vi "Chair Plugin.vi"(10 "DC File":path, 11 "Data IN":T3={"Impulse Positions"=[{"Start"=3107, "End"=3217, "Impulse Plane"=enum."Yaw", "Impulse Direction +ve?"=FALSE, "Time offset"=0, "Amplitude offset"=0.0}, {"Start"=3536, "End"=3646, "Impulse Plane"=enum."Yaw", "Impulse Direction +ve?"=FALSE, "Time offset"=0, "Amplitude offset"=0.0}, {"Start"=4980, "End"=5091, "Impulse Plane"=enum."Yaw", "Impulse Direction +ve?"=TRUE, "Time offset"=0, "Amplitude offset"=0.0}, {"Start"=5459, "End"=5570, "Impulse Plane"=enum."Yaw", "Impulse Direction +ve?"=TRUE, "Time offset"=0, "Amplitude offset"=0.0}, {"Start"=6047, "End"=6157, "Impulse Plane"=enum."Yaw", "Impulse Direction +ve?"=TRUE, "Time offset"=0, "Amplitude offset"=0.0}, {"Start"=6820, "End"=6931, "Impulse Plane"=enum."Yaw", "Impulse Direction +ve?"=TRUE, "Time offset"=0, "Amplitude offset"=0.0}, {"Start"=7337, "End"=7447, "Impulse Plane"=enum."Yaw", "Impulse Direction +ve?"=FALSE, "Time offset"=0, "Amplitude offset"=0.0}, {"Start"=7787, "End"=7897, "Impulse Plane"=enum."Yaw", "Impulse Direction +ve?"=FALSE, "Time offset"=0, "Amplitude offset"=0.0}, {"Start"=8584, "End"=8694, "Impulse Plane"=enum."Yaw", "Impulse Direction +ve?"=FALSE, "Time offset"=0, "Amplitude offset"=0.0}, {"Start"=10739, "End"=10849, "Impulse Plane"=enum."Yaw", "Impulse Direction +ve?"=TRUE, "Time offset"=0, "Amplitude offset"=0.0}, {"Start"=13129, "End"=13240, "Impulse Plane"=enum."Yaw", "Impulse Direction +ve?"=FALSE, "Time offset"=0, "Amplitude offset"=0.0}, {"Start"=13282, "End"=13390, "Impulse Plane"=enum."Yaw", "Impulse Direction +ve?"=FALSE, "Time offset"=0, "Amplitude offset"=0.0}, {"Start"=14766, "End"=14875, "Impulse Plane"=enum."Yaw", "Impulse Direction +ve?"=TRUE, "Time offset"=0, "Amplitude offset"=0.0}, {"Start"=15667, "End"=15777, "Impulse Plane"=enum."Yaw", "Impulse Direction +ve?"=FALSE, "Time offset"=0, "Amplitude offset"=0.0}], "No. Imp"=8, "Parameter Time Series"=[{"time offset"=0.0, "Offset"=0.0, "Gain"=1.0, "inverse"=FALSE, "filter data"=FALSE, "dots"=FALSE, "interpolate"=FALSE, "List 1"=1, "Color Box"=65295, "Boolean"=TRUE}, {"time offset"=0.0, "Offset"=0.0, "Gain"=1.0, "inverse"=FALSE, "filter data"=FALSE, "dots"=FALSE, "interpolate"=FALSE, "List 1"=13, "Color Box"=29695, "Boolean"=TRUE}, {"time offset"=0.0, "Offset"=0.0, "Gain"=1.0, "inverse"=FALSE, "filter data"=FALSE, "dots"=FALSE, "interpolate"=FALSE, "List 1"=21, "Color Box"=16711680, "Boolean"=TRUE}], "Parameter Impuls Series"=[{"Color"=4652800, "Visible"=TRUE, "Channel"=1, "Invert"=FALSE, "Desaccade"=FALSE, "Offset"=0.0, "Gain"=1.0}, {"Color"=16860, "Visible"=TRUE, "Channel"=13, "Invert"=FALSE, "Desaccade"=FALSE, "Offset"=0.0, "Gain"=1.0}, {"Color"=16711680, "Visible"=TRUE, "Channel"=21, "Invert"=FALSE, "Desaccade"=FALSE, "Offset"=0.0, "Gain"=1.0}], "Experiment Parameters"={"Freq"=nan, "Vel"=-1, "Acc"=0, "Stimulus"="Head Impulse -Horizontal"}, "Autosort File"=refnum, "Data File"={"Data Channels"=array22x16587[364914 elements], "Sample Rate"=221, "Channel List"=["-", "Hz Velocity-in-Head", "-", "Hy Velocity-in-Head", "-", "Hx Velocity-in-Head", "-", "-", "-", "-", "-", "Lx Velocity-in-Head", "Ly Velocity-in-Head", "Lz Velocity-in-Head", "-", "-", "-", "-", "-", "Rx Velocity-in-Head", "Ry Velocity-in-Head", "Rz Velocity-in-Head"]}, "Experiment data path"=path "C:/Users/w.figtree/Desktop/Test Data/D246 - Lyndall Westman", "Image data path"=path "C:/Users/w.figtree/Desktop", "LVS data path"=path "/Macintosh HD/Users/patrick/Studium/Diploma Thesis/Data Analysis", "Raw copy path"=path "/Macintosh HD/Users/patrick/Studium/Diploma Thesis/Data Analysis", "filename"="p00195s001e016c001t001.mat", "desaccading parameters"={"Tolerance"=3, "Acc Range"=7000.0, "Sample Rate"=221, "Impulse Plane 2"=enum."Yaw", "Impulse dir"=TRUE}, "Experiment Parameters 2"={"Subject"="Westman Lyndall", "Strain"="(4a) _ OptKin_50_left", "Rotation plane"="", "Experimenter"="Musterdoc", "Trial"=0.0, "Time"=0.0}, "Excel"={"Excel._Application"=refnum, "Use Excel"=TRUE, "Worksheet SINE"=refnum, "Row SINE"=0, "Worksheet TRANS"=refnum, "Row TRANS"=0}, "Session Config File"=refnum, "Autosort Parameter Set"=10, "EMA Version"="EMA 2011b", "desacc "={"Threshold 1 [Acc]"=7000.0, "Threshold 2 [% of TH1]"=60, "tolerance"=3, "Search WD "=0.1, " always use TH2"=FALSE, "Range"=3.0, "Max time"=120.0, "Min time"=20.0, "Velocity Threshold"=150}, "Cycle Nr for Saccades"={"POS"=0, "NEG"=6}, "calibration name"="No file selected"} {"Parameter Time Series"."time offset" format="%.3f"; "Parameter Time Series"."Gain" format="%.1f"; "Parameter Time Series"."Offset" format="%.1f"; "Parameter Time Series"."List 1" items=["Motor-Pos", "Motor-Vel", "Lx Position-in-Head", "Ly Position-in-Head", "Lz Position-in-Head", "Lx Velocity-in-Head", "Ly Velocity-in-Head", "Lz Velocity-in-Head", "Ll Velocity-in-Head", "Lr Velocity-in-Head", "Lx Accel-in-Head", "Ly Accel-in-Head", "Lz Accel-in-Head", "Rx Position-in-Head", "Ry Position-in-Head", "Rz Position-in-Head", "Rx Velocity-in-Head", "Ry Velocity-in-Head", "Rz Velocity-in-Head", "Rl Velocity-in-Head", "Rr Velocity-in-Head", "Rx Accel-in-Head", "Ry Accel-in-Head", "Rz Accel-in-Head", "Global Trigger", "", "", ""]; "Parameter Impuls Series"."Gain" format="%.1f"; "Parameter Impuls Series"."Offset" format="%.1f"}) -> (2 "Cancelled":bool=TRUE, 3 "Data OUT":T3={"Impulse Positions"=[{"Start"=3107, "End"=3217, "Impulse Plane"=enum."Yaw", "Impulse Direction +ve?"=FALSE, "Time offset"=0, "Amplitude offset"=0.0}, {"Start"=3536, "End"=3646, "Impulse Plane"=enum."Yaw", "Impulse Direction +ve?"=FALSE, "Time offset"=0, "Amplitude offset"=0.0}, {"Start"=4980, "End"=5091, "Impulse Plane"=enum."Yaw", "Impulse Direction +ve?"=TRUE, "Time offset"=0, "Amplitude offset"=0.0}, {"Start"=5459, "End"=5570, "Impulse Plane"=enum."Yaw", "Impulse Direction +ve?"=TRUE, "Time offset"=0, "Amplitude offset"=0.0}, {"Start"=6047, "End"=6157, "Impulse Plane"=enum."Yaw", "Impulse Direction +ve?"=TRUE, "Time offset"=0, "Amplitude offset"=0.0}, {"Start"=6820, "End"=6931, "Impulse Plane"=enum."Yaw", "Impulse Direction +ve?"=TRUE, "Time offset"=0, "Amplitude offset"=0.0}, {"Start"=7337, "End"=7447, "Impulse Plane"=enum."Yaw", "Impulse Direction +ve?"=FALSE, "Time offset"=0, "Amplitude offset"=0.0}, {"Start"=7787, "End"=7897, "Impulse Plane"=enum."Yaw", "Impulse Direction +ve?"=FALSE, "Time offset"=0, "Amplitude offset"=0.0}, {"Start"=8584, "End"=8694, "Impulse Plane"=enum."Yaw", "Impulse Direction +ve?"=FALSE, "Time offset"=0, "Amplitude offset"=0.0}, {"Start"=10739, "End"=10849, "Impulse Plane"=enum."Yaw", "Impulse Direction +ve?"=TRUE, "Time offset"=0, "Amplitude offset"=0.0}, {"Start"=13129, "End"=13240, "Impulse Plane"=enum."Yaw", "Impulse Direction +ve?"=FALSE, "Time offset"=0, "Amplitude offset"=0.0}, {"Start"=13282, "End"=13390, "Impulse Plane"=enum."Yaw", "Impulse Direction +ve?"=FALSE, "Time offset"=0, "Amplitude offset"=0.0}, {"Start"=14766, "End"=14875, "Impulse Plane"=enum."Yaw", "Impulse Direction +ve?"=TRUE, "Time offset"=0, "Amplitude offset"=0.0}, {"Start"=15667, "End"=15777, "Impulse Plane"=enum."Yaw", "Impulse Direction +ve?"=FALSE, "Time offset"=0, "Amplitude offset"=0.0}], "No. Imp"=8, "Parameter Time Series"=[{"time offset"=0.0, "Offset"=0.0, "Gain"=1.0, "inverse"=FALSE, "filter data"=FALSE, "dots"=FALSE, "interpolate"=FALSE, "List 1"=1, "Color Box"=65295, "Boolean"=TRUE}, {"time offset"=0.0, "Offset"=0.0, "Gain"=1.0, "inverse"=FALSE, "filter data"=FALSE, "dots"=FALSE, "interpolate"=FALSE, "List 1"=13, "Color Box"=29695, "Boolean"=TRUE}, {"time offset"=0.0, "Offset"=0.0, "Gain"=1.0, "inverse"=FALSE, "filter data"=FALSE, "dots"=FALSE, "interpolate"=FALSE, "List 1"=21, "Color Box"=16711680, "Boolean"=TRUE}], "Parameter Impuls Series"=[{"Color"=4652800, "Visible"=TRUE, "Channel"=1, "Invert"=FALSE, "Desaccade"=FALSE, "Offset"=0.0, "Gain"=1.0}, {"Color"=16860, "Visible"=TRUE, "Channel"=13, "Invert"=FALSE, "Desaccade"=FALSE, "Offset"=0.0, "Gain"=1.0}, {"Color"=16711680, "Visible"=TRUE, "Channel"=21, "Invert"=FALSE, "Desaccade"=FALSE, "Offset"=0.0, "Gain"=1.0}], "Experiment Parameters"={"Freq"=nan, "Vel"=-1, "Acc"=0, "Stimulus"="Head Impulse -Horizontal"}, "Autosort File"=refnum, "Data File"={"Data Channels"=array22x16587[364914 elements], "Sample Rate"=221, "Channel List"=["-", "Hz Velocity-in-Head", "-", "Hy Velocity-in-Head", "-", "Hx Velocity-in-Head", "-", "-", "-", "-", "-", "Lx Velocity-in-Head", "Ly Velocity-in-Head", "Lz Velocity-in-Head", "-", "-", "-", "-", "-", "Rx Velocity-in-Head", "Ry Velocity-in-Head", "Rz Velocity-in-Head"]}, "Experiment data path"=path "C:/Users/w.figtree/Desktop/Test Data/D246 - Lyndall Westman", "Image data path"=path "C:/Users/w.figtree/Desktop", "LVS data path"=path "/Macintosh HD/Users/patrick/Studium/Diploma Thesis/Data Analysis", "Raw copy path"=path "/Macintosh HD/Users/patrick/Studium/Diploma Thesis/Data Analysis", "filename"="p00195s001e016c001t001.mat", "desaccading parameters"={"Tolerance"=3, "Acc Range"=7000.0, "Sample Rate"=221, "Impulse Plane 2"=enum."Yaw", "Impulse dir"=TRUE}, "Experiment Parameters 2"={"Subject"="Westman Lyndall", "Strain"="(4a) _ OptKin_50_left", "Rotation plane"="", "Experimenter"="Musterdoc", "Trial"=0.0, "Time"=0.0}, "Excel"={"Excel._Application"=refnum, "Use Excel"=TRUE, "Worksheet SINE"=refnum, "Row SINE"=0, "Worksheet TRANS"=refnum, "Row TRANS"=0}, "Session Config File"=refnum, "Autosort Parameter Set"=10, "EMA Version"="EMA 2011b", "desacc "={"Threshold 1 [Acc]"=7000.0, "Threshold 2 [% of TH1]"=60, "tolerance"=3, "Search WD "=0.1, " always use TH2"=FALSE, "Range"=3.0, "Max time"=120.0, "Min time"=20.0, "Velocity Threshold"=150}, "Cycle Nr for Saccades"={"POS"=0, "NEG"=6}, "calibration name"="No file selected"} {"Parameter Time Series"."time offset" format="%.3f"; "Parameter Time Series"."Gain" format="%.1f"; "Parameter Time Series"."Offset" format="%.1f"; "Parameter Time Series"."List 1" items=["Motor-Pos", "Motor-Vel", "Lx Position-in-Head", "Ly Position-in-Head", "Lz Position-in-Head", "Lx Velocity-in-Head", "Ly Velocity-in-Head", "Lz Velocity-in-Head", "Ll Velocity-in-Head", "Lr Velocity-in-Head", "Lx Accel-in-Head", "Ly Accel-in-Head", "Lz Accel-in-Head", "Rx Position-in-Head", "Ry Position-in-Head", "Rz Position-in-Head", "Rx Velocity-in-Head", "Ry Velocity-in-Head", "Rz Velocity-in-Head", "Rl Velocity-in-Head", "Rr Velocity-in-Head", "Rx Accel-in-Head", "Ry Accel-in-Head", "Rz Accel-in-Head", "Global Trigger", "", "", ""]; "Parameter Impuls Series"."Gain" format="%.1f"; "Parameter Impuls Series"."Offset" format="%.1f"})   [LabVIEW 2016]
uses:
  core/type-defs/TD_Statemachine-Data.ctl
  core/type-defs/TD_Time Series.ctl
  core/type-defs/TD_Impulse Parameter.ctl
  <vilib>/Utility/file.llb/Read From Spreadsheet File (DBL).vi
  <userlib>/_OpenG.lib/array/array.llb/Reverse 2D Array (DBL)__ogtk.vi
  core/core.lvlib
panel:
  in  "stop 2":bool
  in  "process":bool
  in  "Tab Control":enum32{"Time Plot", "Impuls Plot"}(tab)
  in  "Plot Selection":T1=[{"time offset"=0.0, "Offset"=0.0, "Gain"=1.0, "inverse"=FALSE, "filter data"=FALSE, "dots"=FALSE, "interpolate"=FALSE, "List 1"=1, "Color Box"=65309, "Boolean"=TRUE}, {"time offset"=0.0, "Offset"=0.0, "Gain"=1.0, "inverse"=FALSE, "filter data"=FALSE, "dots"=FALSE, "interpolate"=FALSE, "List 1"=8, "Color Box"=29695, "Boolean"=TRUE}, {"time offset"=0.0, "Offset"=0.0, "Gain"=1.0, "inverse"=FALSE, "filter data"=FALSE, "dots"=FALSE, "interpolate"=FALSE, "List 1"=14, "Color Box"=16711680, "Boolean"=TRUE}] {"time offset" format="%.3f"; "Gain" format="%.1f"; "Offset" format="%.1f"; "List 1" items=["Chair Position", "Chair Velocity", "Light Off/On", "Lx Position-in-Head", "Ly Position-in-Head", "Lz Position-in-Head", "Lx Velocity-in-Head", "Ly Velocity-in-Head", "Lz Velocity-in-Head", "Rx Position-in-Head", "Ry Position-in-Head", "Rz Position-in-Head", "Rx Velocity-in-Head", "Ry Velocity-in-Head", "Rz Velocity-in-Head"]}
  in  "Plot Selection 2":T2=[{"Color"=4652800, "Visible"=TRUE, "Channel"=1, "Invert"=FALSE, "Desaccade"=FALSE, "Offset"=0.0, "Gain"=1.0}, {"Color"=29695, "Visible"=TRUE, "Channel"=8, "Invert"=FALSE, "Desaccade"=FALSE, "Offset"=0.0, "Gain"=1.0}, {"Color"=16711680, "Visible"=TRUE, "Channel"=14, "Invert"=FALSE, "Desaccade"=FALSE, "Offset"=0.0, "Gain"=1.0}] {"Gain" format="%.1f"; "Offset" format="%.1f"; "Channel" items=["Chair Position", "Chair Velocity", "Light Off/On", "Lx Position-in-Head", "Ly Position-in-Head", "Lz Position-in-Head", "Lx Velocity-in-Head", "Ly Velocity-in-Head", "Lz Velocity-in-Head", "Rx Position-in-Head", "Ry Position-in-Head", "Rz Position-in-Head", "Rx Velocity-in-Head", "Ry Velocity-in-Head", "Rz Velocity-in-Head"]}
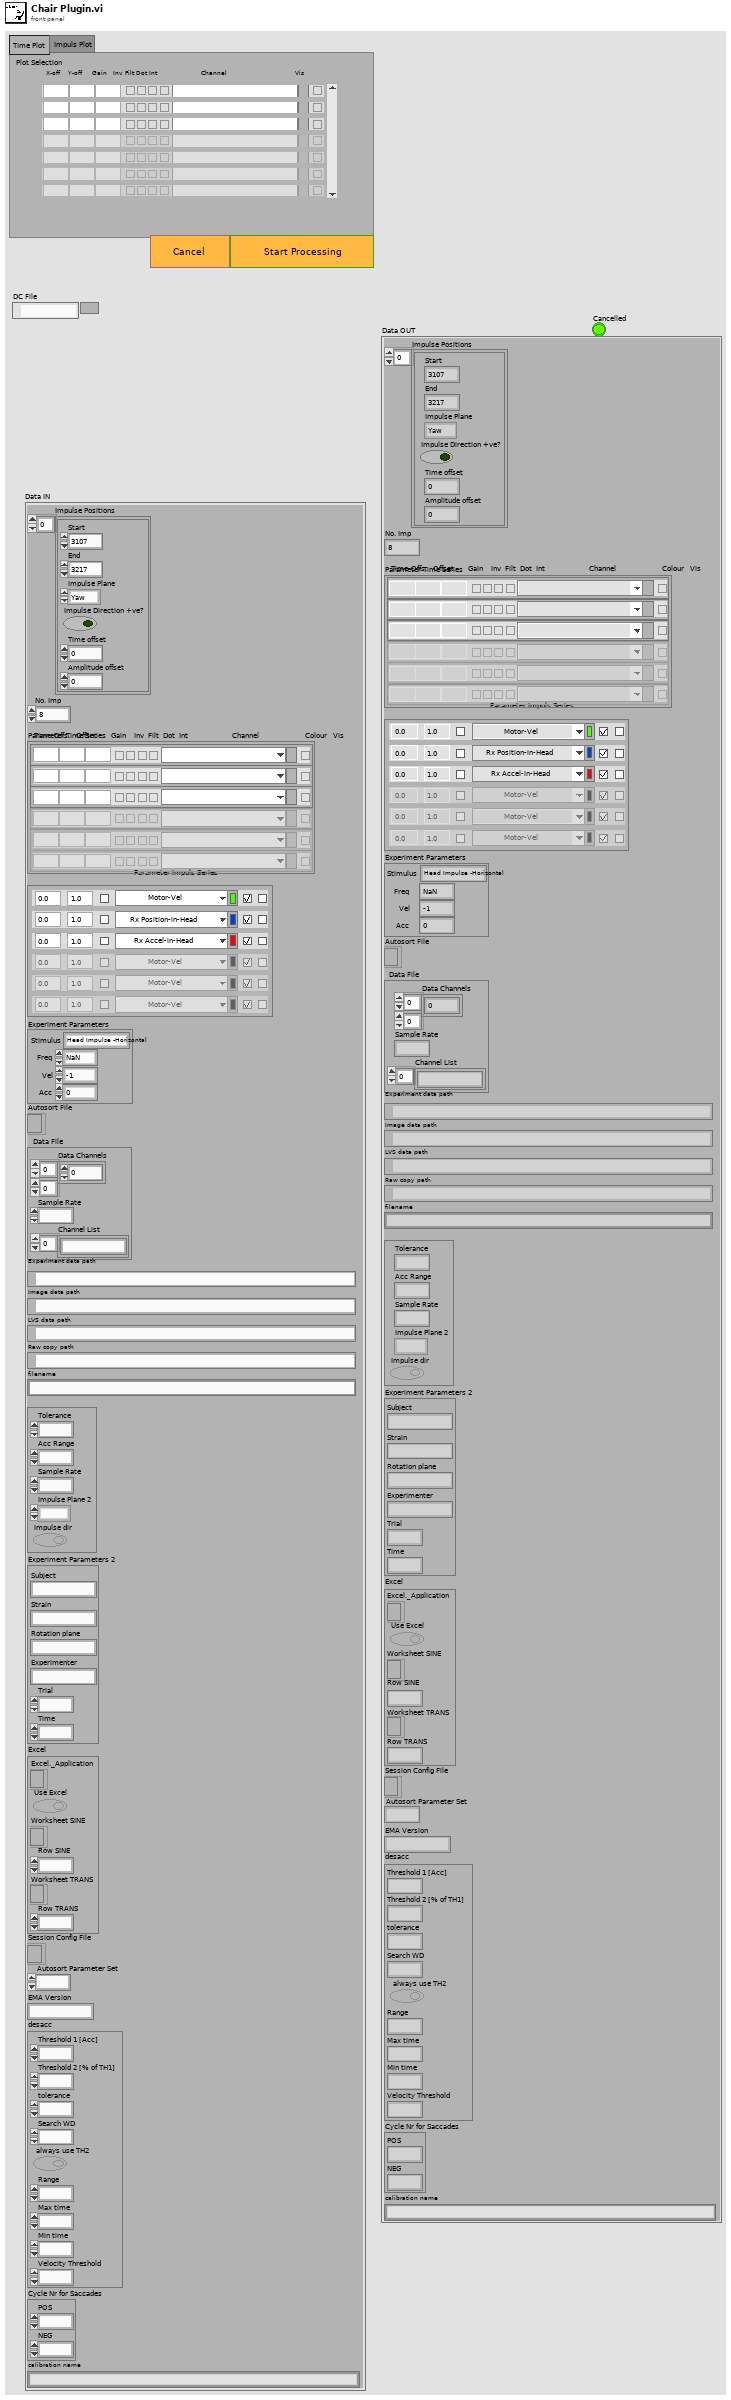
[diagram p1: front panel]
types:
  T1 = typedef "core.lvlib/TD_Time Series.ctl" = cluster{"time offset":dbl, "Offset":dbl, "Gain":dbl, "inverse":bool, "filter data":bool, "dots":bool, "interpolate":bool, "List 1":u16, "Color Box":u32, "Boolean":bool}[]
  T2 = typedef "core.lvlib/TD_Impulse Parameter.ctl" = cluster{"Color":u32, "Visible":bool, "Channel":u16, "Invert":bool, "Desaccade":bool, "Offset":dbl, "Gain":dbl}[]
  T3 = typedef "core.lvlib/TD_Statemachine-Data.ctl" = cluster{"Impulse Positions":cluster{"Start":i32, "End":i32, "Impulse Plane":enum16{"Other", "Yaw", "Pitch", "Roll", "LARP", "RALP"}, "Impulse Direction +ve?":bool, "Time offset":i32, "Amplitude offset":dbl}[], "No. Imp":i32, "Parameter Time Series":T1, "Parameter Impuls Series":T2, "Experiment Parameters":cluster{"Freq":dbl, "Vel":i32, "Acc":i32, "Stimulus":string}, "Autosort File":refnum<file>, "Data File":cluster{"Data Channels":dbl[][], "Sample Rate":i32, "Channel List":string[]}, "Experiment data path":path, "Image data path":path, "LVS data path":path, "Raw copy path":path, "filename":string, "desaccading parameters":cluster{"Tolerance":i32, "Acc Range":dbl, "Sample Rate":i32, "Impulse Plane 2":enum16{"Other", "Yaw", "Pitch", "Roll", "LARP", "RALP"}, "Impulse dir":bool}, "Experiment Parameters 2":cluster{"Subject":string, "Strain":string, "Rotation plane":string, "Experimenter":string, "Trial":dbl, "Time":dbl}, "Excel":cluster{"Excel._Application":refnum<k7>, "Use Excel":bool, "Worksheet SINE":refnum<k7>, "Row SINE":i32, "Worksheet TRANS":refnum<k7>, "Row TRANS":i32}, "Session Config File":refnum<file>, "Autosort Parameter Set":i32, "EMA Version":string, "desacc ":cluster{"Threshold 1 [Acc]":dbl, "Threshold 2 [% of TH1]":i32, "tolerance":i32, "Search WD ":dbl, " always use TH2":bool, "Range":dbl, "Max time":dbl, "Min time":dbl, "Velocity Threshold":i32}, "Cycle Nr for Saccades":cluster{"POS":i32, "NEG":i32}, "calibration name":string}
  T4 = cluster{"File Path":path, "Raw Data":sgl[][], "Sample Rate":i32}
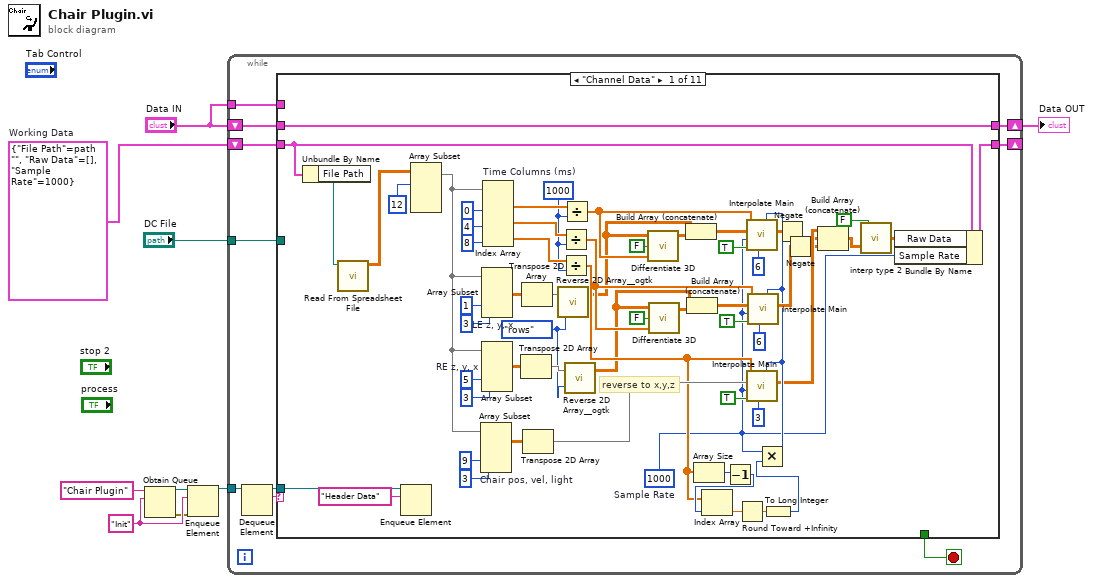
[diagram p0: block diagram]
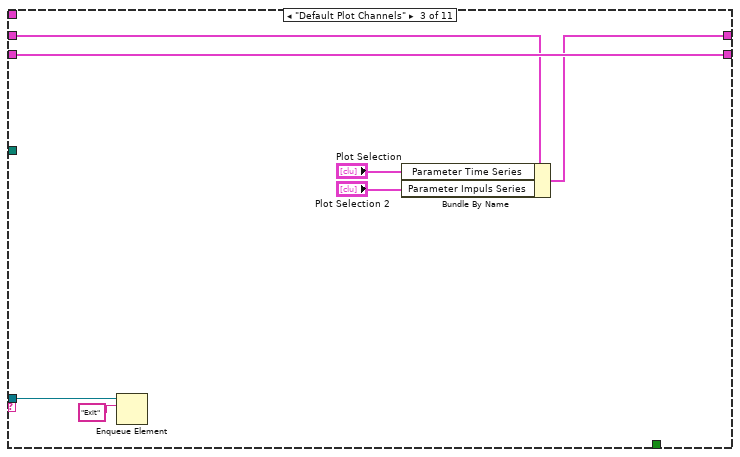
[diagram p3: hidden frame]
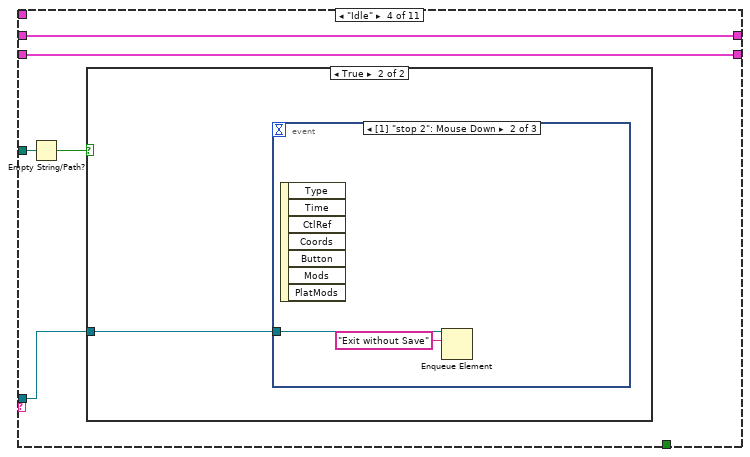
[diagram p4: hidden frame]
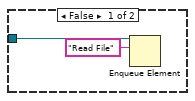
[diagram p5: hidden frame]
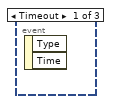
[diagram p6: hidden frame]
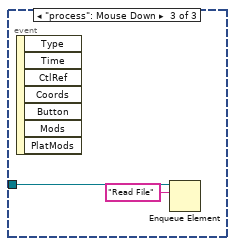
[diagram p7: hidden frame]
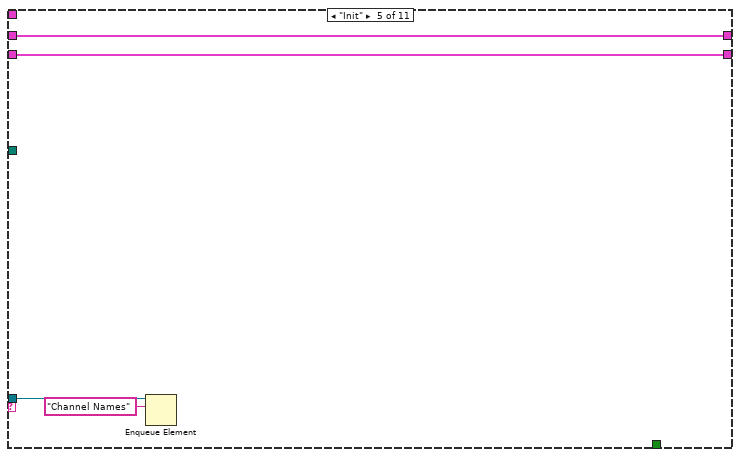
[diagram p8: hidden frame]
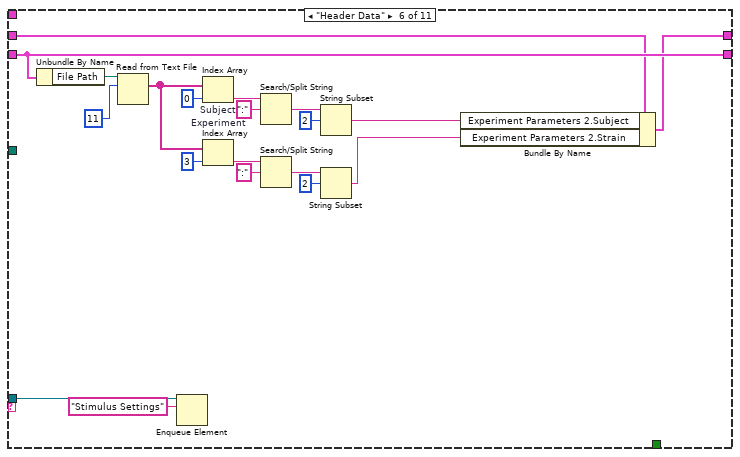
[diagram p9: hidden frame]
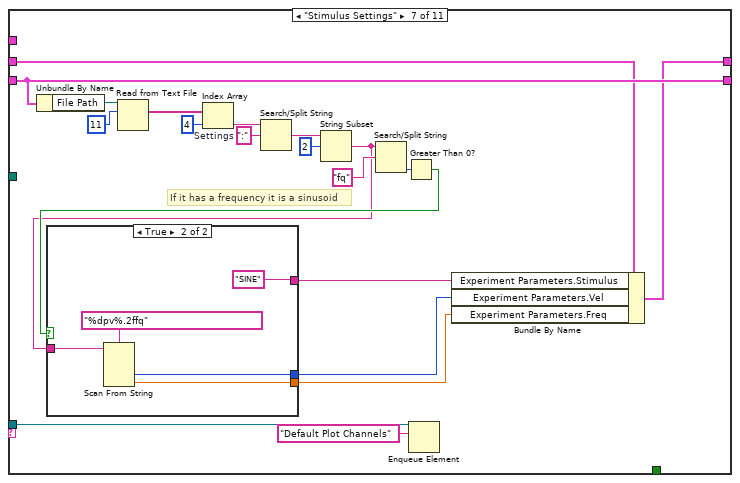
[diagram p10: hidden frame]
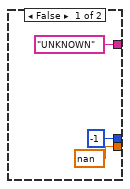
[diagram p11: hidden frame]
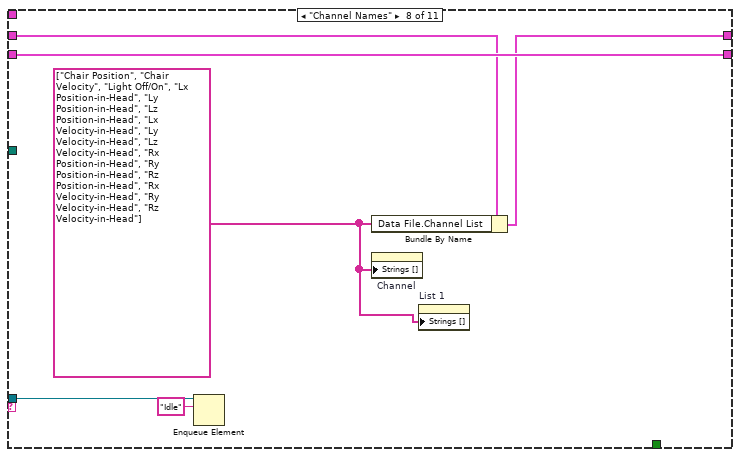
[diagram p12: hidden frame]
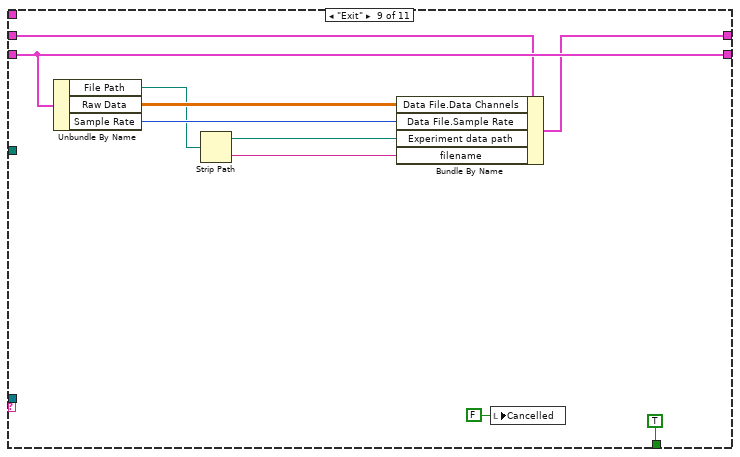
[diagram p13: hidden frame]
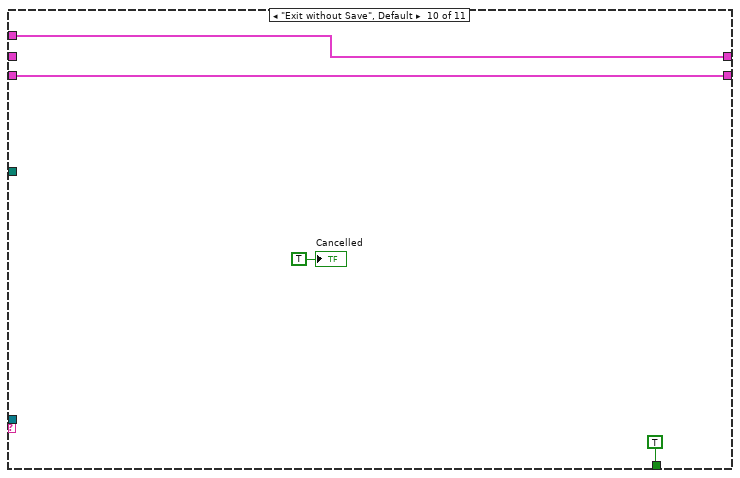
[diagram p14: hidden frame]
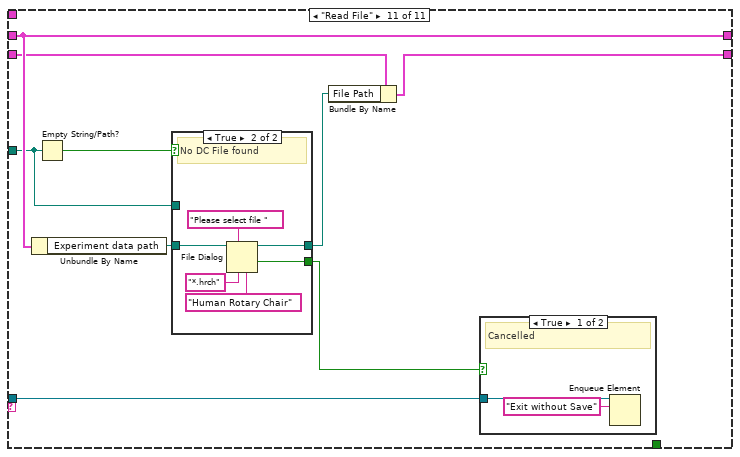
[diagram p15: hidden frame]
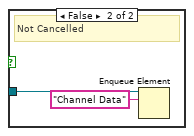
[diagram p16: hidden frame]
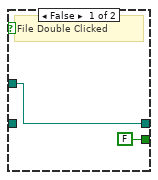
[diagram p17: hidden frame]
diagram:
  w2 = T4 {"File Path"=path "", "Raw Data"=[], "Sample Rate"=1000}  # Working Data
  w7 = "Init" ("name (unnamed)")
  n1 = Obtain Queue(name (unnamed)="Chair Plugin", element data type=w7) -> (queue out=w8:refnum<queue>, error out=w6:errorcluster)  [unwired: 3 in, 1 out]
  n2 = Enqueue Element(queue=w8, element=w7, error in (no error)=w6) -> (queue out=w5:refnum<queue>)  [unwired: 1 in, 2 out]
  n3 = while {
    tunnel: w5 -> [w19]
    tunnel: "DC File" -> [w15]
    shift-right: [w16] -> w4
    shift-left: "Data IN" -> [w17]
    shift-right: [w13] -> _
    shift-left: w2 -> [w14]
    tunnel: "Data IN" -> [w10]
    stop <- w11 stop-if-true
    n4 = Dequeue Element(queue=w19) -> (queue out=w12:refnum<queue>, element=w18:string)  [unwired: 2 in, 2 out]
    n5 = case shown="\"Channel Data\"" w18 {
      tunnel: w17 -> [w80 w82 w88 w94 w105 w117 w137 w158 w165 _ w181]
      tunnel: [w80 w82 w87 w94 w105 w116 w136 w157 w164 w172 w181] -> w16
      tunnel: w15 -> [_ _ _ w92 _ _ _ _ _ _ w179]
      tunnel: w14 -> [w35 w81 w89 w93 w104 w125 w145 w159 w168 w171 w177]
      tunnel: [w34 w81 w89 w93 w104 w125 w145 w159 w168 w171 w176] -> w13
      tunnel: w12 -> [w32 _ w84 w90 w103 w107 w127 w156 _ _ w175]
      tunnel: [_ _ _ _ _ _ _ _ TRUE TRUE _] -> w11
      tunnel: w10 -> [_ _ _ _ _ _ _ _ _ w172 _]
      frame "Channel Data" {
        w23 = enum16{"rows", "columns"}."rows" ("by rows or columns (rows)")
        w40 = 1000 ("Sample Rate")
        w33 = 1000  # Sample Rate
        # "reverse to x,y,z"
        n6 = Unbundle By Name(w35) -> ("File Path"=w36:path)
        n7 = call-poly <vilib>:"Read From Spreadsheet File.vi"("file path (dialog if empty)"=w36) -> ("all rows"=w78:dbl[][])  [unwired: 6 in, 4 out]
        n8 = Enqueue Element(queue=w32, element="Header Data") -> ()  [unwired: 2 in, 3 out]
        n9 = Array Subset(array=w78, index (row)=12 ("index")) -> (w63:dbl[][])  [unwired: 3 in]
        n10 = Array Subset "Chair pos, vel, light"(array=w63, index (col)=9 ("index"), length (col)=3 ("length")) -> (w46:dbl[][])  [unwired: 2 in]
        n11 = Array Subset "LE z, y, x"(array=w63, index (col)=1 ("index"), length (col)=3 ("length")) -> (w71:dbl[][])  [unwired: 2 in]
        n12 = Array Subset "RE z, y, x"(array=w63, index (col)=5 ("index"), length (col)=3 ("length")) -> (w66:dbl[][])  [unwired: 2 in]
        n13 = Index Array "Time Columns (ms)"(array=w63, index (col) #1=0 ("index (row)"), index (col) #2=4 ("index (row)"), index (col) #3=8 ("index (row)")) -> (element #1=w43:dbl[], element #2=w42:dbl[], element #3=w41:dbl[])  [unwired: 3 in]
        n14 = Transpose 2D Array(2D array=w66) -> (transposed array=w25:dbl[][])
        n15 = Transpose 2D Array(2D array=w71) -> (transposed array=w27:dbl[][])
        n16 = Transpose 2D Array(2D array=w46) -> (transposed array=w45:dbl[][])
        n17 = call-poly <userlib>:"Reverse 2D Array__ogtk.vi"("by rows or columns (rows)"=w23, "Array"=w27) -> ("Reversed Array"=w26:dbl[][])  [unwired: 1 in]
        n18 = Divide(x=w42, y=w40) -> (x/y=w38:dbl[])
        n19 = Divide(x=w41, y=w40) -> (x/y=w39:dbl[])
        n20 = Divide(x=w43, y=w40) -> (x/y=w37:dbl[])
        n21 = call-poly <userlib>:"Reverse 2D Array__ogtk.vi"("by rows or columns (rows)"=w23, "Array"=w25) -> ("Reversed Array"=w24:dbl[][])  [unwired: 1 in]
        n22 = call "Differentiate 3D.vi"("Timebase"=w37, "Fixed Sample Rate"=FALSE, "Data (in)"=w26) -> ("Data (differentiated)"=w72:dbl[][])  [unwired: 2 in]
        n23 = call "Differentiate 3D.vi"("Timebase"=w38, "Fixed Sample Rate"=FALSE, "Data (in)"=w24) -> ("Data (differentiated)"=w67:dbl[][])  [unwired: 2 in]
        n24 = Build Array (concatenate)(w26, w72) -> (w70:dbl[][])
        n25 = Build Array (concatenate)(w24, w67) -> (w69:dbl[][])
        n26 = Array Size(array=w39) -> (size(s)=w56:i32)
        n27 = Decrement(x=w56) -> (x-1=w44:i32)
        n28 = Index Array(array=w39, index=w44) -> (element=w55:dbl)
        n29 = Round Toward +Infinity(x=w55) -> (ceil(x): smallest int >= x=w54:dbl)
        n30 = To Long Integer(number=w54) -> (32bit integer=w50:i32)
        n31 = Multiply(x=w33, y=w50) -> (x*y=w51:i32)
        n32 = call "Interpolate Main.vi"("Length"=w51, "Data Channels"=6, "NaN"=TRUE, "Sample Rate"=w33, "Data"=w70, "Time"=w37) -> ("Interp Data"=w53:dbl[][])  [unwired: 4 in]
        n33 = call "Interpolate Main.vi"("Length"=w51, "Data Channels"=3, "NaN"=TRUE, "Sample Rate"=w33, "Data"=w45, "Time"=w39) -> ("Interp Data"=w28:dbl[][])  [unwired: 4 in]
        n34 = call "Interpolate Main.vi"("Length"=w51, "Data Channels"=6, "NaN"=TRUE, "Sample Rate"=w33, "Data"=w69, "Time"=w38) -> ("Interp Data"=w52:dbl[][])  [unwired: 4 in]
        n35 = Negate(x=w53) -> (-x=w21:dbl[][])
        n36 = Negate(x=w52) -> (-x=w22:dbl[][])
        n37 = Build Array (concatenate)(w28, w21, w22) -> (w30:dbl[][])
        n38 = call "interp type 2.vi"("NaN"=w30, "Remove front and end"=FALSE) -> ("Interpolated"=w29:dbl[][])
        n39 = Bundle By Name(cluster=w35, "Raw Data"=w29, "Sample Rate"=w33) -> (w34:T4)
      }
      frame "Template" {
      }
      frame "Default Plot Channels" {
        n40 = Enqueue Element(queue=w84, element="Exit") -> ()  [unwired: 2 in, 3 out]
        n41 = Bundle By Name(cluster=w88, "Parameter Time Series"="Plot Selection", "Parameter Impuls Series"="Plot Selection 2") -> (w87:T3)
      }
      frame "Idle" {
        n42 = Empty String/Path?(string/path=w92) -> (empty?=w91:bool)
        n43 = case shown="True" w91 {
          tunnel: w90 -> [w96 w97]
          frame False {
            n44 = Enqueue Element(queue=w96, element="Read File") -> ()  [unwired: 2 in, 3 out]
          }
          frame True {
            n45 = event shown="[1] \"stop 2\": Mouse Down" {
              selector: _ -> [_ _ _]
              dyn-events: _ -> [_ _ _]
              timeout: _ -> [_ _ _]
              tunnel: w97 -> [_ w99 w101]
              event Timeout {
                n46 = event-data() -> ()  [unwired: 1 in, 2 out]
              }
              event "stop 2": Mouse Down {
                n47 = event-data() -> ()  [unwired: 1 in, 7 out]
                n48 = Enqueue Element(queue=w99, element="Exit without Save") -> ()  [unwired: 2 in, 3 out]
              }
              event "process": Mouse Down {
                n49 = event-data() -> ()  [unwired: 1 in, 7 out]
                n50 = Enqueue Element(queue=w101, element="Read File") -> ()  [unwired: 2 in, 3 out]
              }
            }
          }
        }
      }
      frame "Init" {
        n51 = Enqueue Element(queue=w103, element="Channel Names") -> ()  [unwired: 2 in, 3 out]
      }
      frame "Header Data" {
        n52 = Unbundle By Name(w125) -> ("File Path"=w124:path)
        n53 = Read from Text File(file (use dialog)=w124, count=11) -> (text=w109:string[])  [unwired: 2 in, 3 out]
        n54 = Enqueue Element(queue=w107, element="Stimulus Settings") -> ()  [unwired: 2 in, 3 out]
        n55 = Index Array "Subject"(array=w109, index=0) -> (element=w121:string)
        n56 = Index Array "Experiment"(array=w109, index=3) -> (element=w111:string)
        n57 = Search/Split String(string=w121, search string/char (-)=":") -> (match + rest of string=w118:string)  [unwired: 1 in, 2 out]
        n58 = Search/Split String(string=w111, search string/char (-)=":") -> (match + rest of string=w114:string)  [unwired: 1 in, 2 out]
        n59 = String Subset(string=w118, offset (0)=2) -> (substring=w115:string)  [unwired: 1 in]
        n60 = String Subset(string=w114, offset (0)=2) -> (substring=w108:string)  [unwired: 1 in]
        n61 = Bundle By Name(cluster=w117, "Experiment Parameters 2.Subject"=w115, "Experiment Parameters 2.Strain"=w108) -> (w116:T3)
      }
      frame "Stimulus Settings" {
        # "If it has a frequency it is a sinusoid"
        n62 = Unbundle By Name(w145) -> ("File Path"=w144:path)
        n63 = Read from Text File(file (use dialog)=w144, count=11) -> (text=w135:string[])  [unwired: 2 in, 3 out]
        n64 = Index Array "Settings"(array=w135, index=4) -> (element=w141:string)
        n65 = Search/Split String(string=w141, search string/char (-)=":") -> (match + rest of string=w138:string)  [unwired: 1 in, 2 out]
        n66 = String Subset(string=w138, offset (0)=2) -> (substring=w131:string)  [unwired: 1 in]
        n67 = Search/Split String(string=w131, search string/char (-)="fq") -> (offset of match=w133:i32)  [unwired: 1 in, 2 out]
        n68 = Greater Than 0?(x=w133) -> (x > 0?=w132:bool)
        n69 = case shown="True" w132 {
          tunnel: w131 -> [_ w153]
          tunnel: [-1 w151] -> w130
          tunnel: [nan w150] -> w129
          tunnel: ["UNKNOWN" "SINE"] -> w128
          frame False {
          }
          frame True {
            n70 = Scan From String(format string="%dpv%.2ffq", input string=w153) -> (output 1=w151:i32, output 2=w150:dbl)  [unwired: 4 in, 3 out]
          }
        }
        n71 = Enqueue Element(queue=w127, element="Default Plot Channels") -> ()  [unwired: 2 in, 3 out]
        n72 = Bundle By Name(cluster=w137, "Experiment Parameters.Stimulus"=w128, "Experiment Parameters.Vel"=w130, "Experiment Parameters.Freq"=w129) -> (w136:T3)
      }
      frame "Channel Names" {
        w154 = string[] ["Chair Position", "Chair Velocity", "Light Off/On", "Lx Position-in-Head", "Ly Position-in-Head", "Lz Position-in-Head", "Lx Velocity-in-Head", "Ly Velocity-in-Head", "Lz Velocity-in-Head", "Rx Position-in-Head", "Ry Position-in-Head", "Rz Position-in-Head", "Rx Velocity-in-Head", "Ry Velocity-in-Head", "Rz Velocity-in-Head"]
        n73 = Enqueue Element(queue=w156, element="Idle") -> ()  [unwired: 2 in, 3 out]
        n74 = Bundle By Name(cluster=w158, "Data File.Channel List"=w154) -> (w157:T3)
        n75 = property on="Channel" class="Ring (strict)"("Strings []"=w154) -> ()  [unwired: 2 in, 2 out]
        n76 = property on="List 1" class="Ring (strict)"("Strings []"=w154) -> ()  [unwired: 2 in, 2 out]
      }
      frame "Exit" {
        n77 = Unbundle By Name(w168) -> ("File Path"=w161:path, "Raw Data"=w167:sgl[][], "Sample Rate"=w166:i32)
        n78 = Strip Path(path=w161) -> (stripped path=w163:path, name=w162:string)
        n79 = Bundle By Name(cluster=w165, "Data File.Data Channels"=w167, "Data File.Sample Rate"=w166, "Experiment data path"=w163, "filename"=w162) -> (w164:T3)
        n80 = local write "Cancelled"(FALSE ("Cancelled")) -> ()
      }
      frame "Exit without Save", Default {
        "Cancelled" <- TRUE
      }
      frame "Read File" {
        n81 = Unbundle By Name(w181) -> ("Experiment data path"=w180:path)
        n82 = Empty String/Path?(string/path=w179) -> (empty?=w182:bool)
        n83 = case shown="True" w182 {
          tunnel: w180 -> [_ w194]
          tunnel: [FALSE ("cancelled") w192] -> w174
          tunnel: w179 -> [w188 _]
          tunnel: [w188 w191] -> w178
          frame False {
            # "File Double Clicked"
          }
          frame True {
            # "No DC File found"
            n84 = File Dialog(4:"Human Rotary Chair" ("pattern label"), 6:"*.hrch" ("pattern (all files)"), 7:"Please select file " ("prompt"), 11:w194) -> (1:w192:bool, 3:w191:path)  [unwired: 3 in, 2 out]
          }
        }
        n85 = Bundle By Name(cluster=w177, "File Path"=w178) -> (w176:T4)
        n86 = case shown="True" w174 {
          tunnel: w175 -> [w184 w186]
          frame True {
            # "Cancelled"
            n87 = Enqueue Element(queue=w184, element="Exit without Save") -> ()  [unwired: 2 in, 3 out]
          }
          frame False {
            # "Not Cancelled"
            n88 = Enqueue Element(queue=w186, element="Channel Data") -> ()  [unwired: 2 in, 3 out]
          }
        }
      }
    }
  }
  "Data OUT" <- w4
